vi "Gyro PID Back Color Assisted.vi"(6 "Target angle":sgl, 7 "Threshold to Stop":i32=1200, 8 "Threshold to slow & check ref.":i32=1000, 9 "Min. speed":i32=20, 10 "Max. speed":i32=40, 11 "EV3 in":T1) -> (3 "EV3 out":T1)   [LabVIEW 2016]
uses:
  <vilib>/NXT/Subs/LVHSConnector.ctl
  <vilib>/NXT/LegoClasses/BrickReference/BrickReference.lvclass
  <vilib>/NXT/Block Support/NXT_OutputPort.ctl
  <vilib>/NXT/Block Support/NXT_InputPort.ctl
  <vilib>/NXT/NXTIO Xnodes/NXTIONodeSubVIs/LEGOResetMotors.vi
  <vilib>/NXT/Dual Mode Library/Motors/Rotation.vi
  <vilib>/NXT/Dual Mode Library/Sensors/EV3_Color_Reflect.vi
  <vilib>/NXT/NXTIO Xnodes/NXTIONodeSubVIs/NXTMotorSteeringOn.vi
  <vilib>/NXT/NXTIO Xnodes/NXTIONodeSubVIs/NXTStopMotors.vi
  <vilib>/NXT/Dual Mode Library/Waits/Wait_Num.vi
  <vilib>/NXT/NXTIO Xnodes/NXTIOXNode/NXTIO.xnode
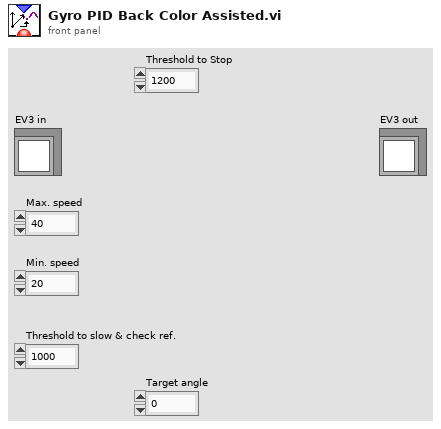
[diagram p1: front panel]
types:
  T1 = typedef "LVHSConnector.ctl" = refnum<class "BrickReference.lvclass">
  T2 = typedef "NXT_OutputPort.ctl" = u8
  T3 = typedef "NXT_InputPort.ctl" = u32
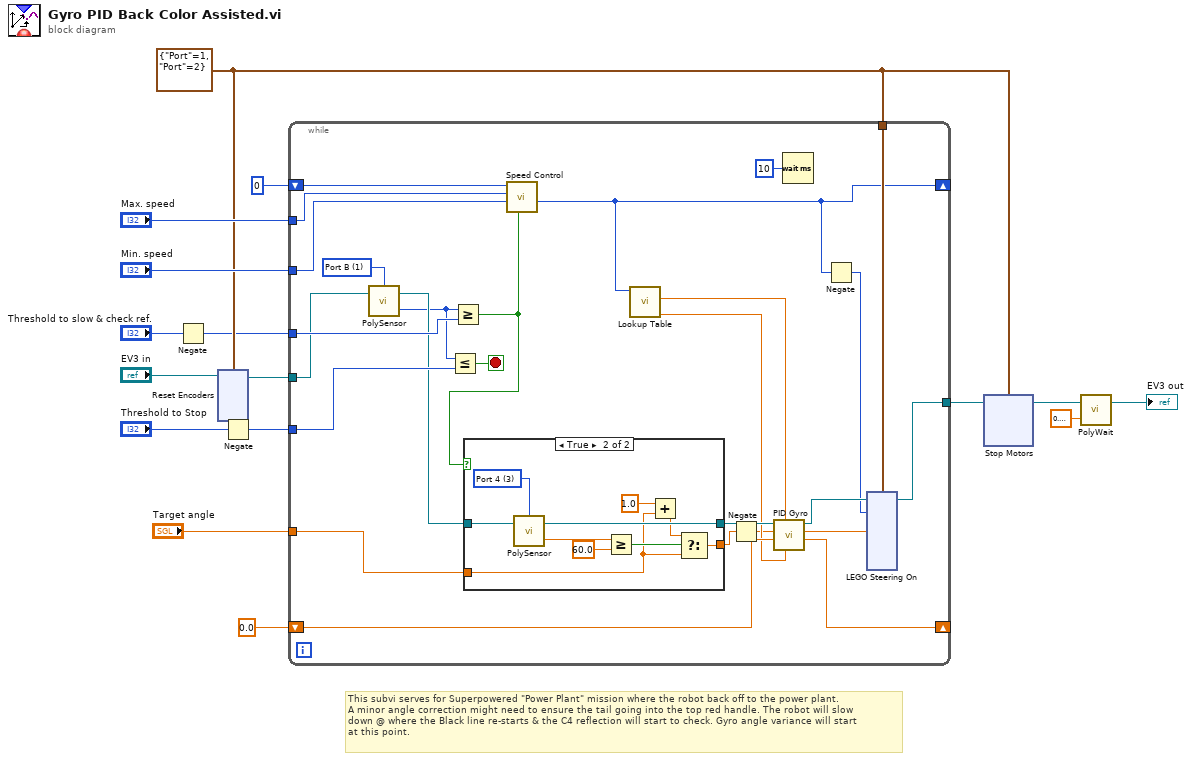
[diagram p0: block diagram]
diagram:
  w6 = cluster{"Port":T2, "Port":T2} {"Port"=1, "Port"=2} ("Motor")
  # "This subvi serves for Superpowered \"Power Plant\" mission where the robot back off to the power plant.\nA minor angle correction might need to ensure the tail going into the top red handle. The robot will slow\ndown @ where the Black line re-starts & the C4 reflection will start to check. Gyro angle variance will start\nat this point."
  n1 = Negate(x="Threshold to slow & check ref.") -> (-x=w2:i32)
  n2 = xnode "Reset Encoders"("Motors"=w6, "NXT/EV3"="EV3 in") -> ("NXT/EV3"=w12:T1)
  n3 = Negate(x="Threshold to Stop") -> (-x=w1:i32)
  n4 = while {
    tunnel: w12 -> [w33]
    shift-right: [w42] -> _
    shift-left: sgl 0.0 -> [w32]
    tunnel: "Target angle" -> [w19]
    tunnel: [w39] -> w8
    tunnel: w6 -> [w41]
    shift-right: [w25] -> _
    shift-left: 0 -> [w37]
    tunnel: "Min. speed" -> [w34]
    tunnel: "Max. speed" -> [w36]
    tunnel: w2 -> [w35]
    tunnel: w1 -> [w31]
    stop <- w27 stop-if-true
    w40 = T2 1 items=["Port A", "Port B", "Port C", "Port D"] ("Port (Port A)")
    n5 = call-poly <vilib>:"PolySensor.vi"("NXT/EV3"=w33, "Port (Port A)"=w40) -> ("Angle of Rotation"=w21:i32, "NXT/EV3"=w30:T1)  [unwired: 1 in]
    n6 = Less Or Equal?(x=w21, y=w31) -> (x <= y?=w27:bool)
    n7 = Greater Or Equal?(x=w21, y=w35) -> (x >= y?=w20:bool)
    n8 = case shown="True" w20 {
      tunnel: w30 -> [w44 w53]
      tunnel: [w44 w52] -> w29
      tunnel: w19 -> [w43 w48]
      tunnel: [w43 w45] -> w18
      frame False {
      }
      frame True {
        w54 = T3 3 items=["Port 1", "Port 2", "Port 3", "Port 4"] ("Port (Port 1)")
        n9 = call-poly <vilib>:"PolySensor.vi"("NXT/EV3"=w53, "Port (Port 1)"=w54) -> ("Scaled Value"=w51:sgl, "NXT/EV3"=w52:T1)  [unwired: 1 in]
        n10 = Greater Or Equal?(x=w51, y=sgl 60.0) -> (x >= y?=w49:bool)
        n11 = Add(x=sgl 1.0, y=w48) -> (x+y=w46:sgl)
        n12 = Select(t=w46, s=w49, f=w48) -> (s? t:f=w45:sgl)
      }
    }
    n13 = call "Speed Control.vi"("Speed Up or Down?"=w20, "Min. speed"=w34, "Max. speed"=w36, "Ini. speed"=w37) -> ("Speed out"=w25:i32)  [unwired: 7 in]
    n14 = call "Lookup Table.vi"("Speed"=w25) -> ("I"=w23:dbl, "P"=w24:dbl)  [unwired: 9 in]
    n15 = Negate(x=w18) -> (-x=w17:sgl)
    n16 = call "PID Gyro.vi"("K_i"=w23, "K_p"=w24, "Previous integral"=w32, "Target angle"=w17, "EV3 in"=w29) -> ("New integral"=w42:sgl, "Total error"=w22:sgl, "EV3 out"=w28:T1)  [unwired: 4 in]
    n17 = Wait (ms)(milliseconds to wait=u32 10) -> ()  [unwired: 1 out]
    n18 = Negate(x=w25) -> (-x=w26:i32)
    n19 = xnode "LEGO Steering On"("Steering 1"=w22, "Power 1"=w26, "Motors"=w41, "NXT/EV3"=w28) -> ("NXT/EV3"=w39:T1)
  }
  n20 = xnode "Stop Motors"("Motors"=w6, "NXT/EV3"=w8) -> ("NXT/EV3"=w7:T1)
  n21 = call-poly <vilib>:"PolyWait.vi"("Time (1 sec)"=sgl 0.2, "NXT/EV3"=w7) -> ("NXT/EV3"=→"EV3 out":T1)  [unwired: 2 in]
